vi "Database.Connect.vi"(8 "error in":errorcluster, 11 "Data in":T1) -> (0 "error out":errorcluster, 3 "Data out":T1)   [LabVIEW 2016]
doc: "Connect to database\n\nWabco 2017 All right reserved\nAuthor: maciej.szupienko@wabco-auto.com"
uses:
  Database.Data.ctl
  Database.Data.Sets.ctl
  Handler/Database.Handler.Data.Status.ctl
  Tools/Translator/Translator.Message.ctl
  Tools/EventLog/EventLog.EventSource.ctl
  Tools/EventLog/EventLog.New(array).vi
  Tools/EventLog/EventLog.CreateError(array).vi
  Tools/ErrorHandling/ErrorHandling.Create.vi
  Global/ApplicationGlobal.vi
  Tools/EventLog/EventLog.Buffer.vi
  Tools/EventLog/EventLog.File.ReadWrite.vi
  Tools/Tma.lib/string.llb/Join array to string.vi
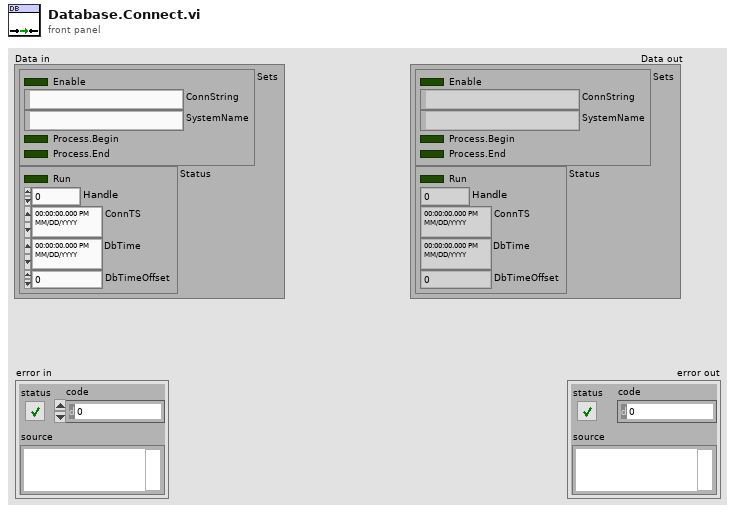
[diagram p1: front panel]
types:
  T1 = typedef "Database.Data.ctl" = cluster{"Sets":T2, "Status":T3}
  T2 = typedef "Database.Data.Sets.ctl" = cluster{"Enable":bool, "ConnString":string, "SystemName":string, "Process.Begin":bool, "Process.End":bool}
  T3 = typedef "Database.Handler.Data.Status.ctl" = cluster{"Run":bool, "Handle":i32, "ConnTS":timestamp, "DbTime":timestamp, "DbTimeOffset":dbl}
  T4 = typedef "EventLog.EventSource.ctl" = enum16{"All", "Gui", "Cache", "PLC1", "PLC2", "PLC3", "DB", "DB01", "DB02", "DB03", "DB04", "DB05", "DB06", "DB07", "DB08", "DB09", "DB10", "DB11", "DB12", "DB13", "DB14", "DB15", "DB16"}
  T5 = typedef "Translator.Message.ctl" = enum16{"-", "Event confirmed", "Log out", "Log in", "Shutdown", "Cancel", "Start", "Continue", "Stop", "On", "Off", "OK", "NOK", "NOK %s", "This", "Prev", "Home", "Work", "In progress...", "Missing", "Empty", "Hardware failure", "Initial", "Error %d >> %s", "Error %d >> %s >> %s", "Starting %s", "Quitting %s", "Configured", "Initializing", "Quitting", "Loading", "Running %s", "Stopped", "Summary", "Do you want to continue?", "Do you want to exit?", "Log out?", "System", "All", "IDLE", "Translating...%s", "Not found", "Alarm %s", "Run", "Skip", "Abort", "Repeat", "Please wait...", "Database disconnected", "Login to database successful", "Login to database failed: %d; %s", "Get process step data for %s", "Changeover off", "Changeover into %s", "Product %s | %s found in cache with status %d at previous station", "Product %s | %s found in database with status %d at previous station", "Product %s | %s not found in cache at previous station", "Product %s | %s not found in database at previous station", "Product %s | %s found in cache with status %d at this station (%d repetion)", "Product %s | %s found in database with status %d at this station (%d repetition)", "Product %s | %s not found in cache at this station", "Product %s | %s not found in database at this station", "Product %s | %s found in cache for component %s | %s", "Product %s | %s found in database for component %s | %s", "Product not found in cache for component %s | %s", "Product not found in database for component %s | %s", "Product %s | %s connected with component %s | %s (cache)", "Product %s | %s connected with component %s | %s (database)", "New data for %s | %s (cache)", "New data for %s | %s (database)", "File %s moved (cache)", "File %s deleted (cache)", "Msg %d >> %s", "PLC LifeBit Failure", "Reconnecting DB", "Reconnecting PLC", "Free disk space is below 1GB - contact technician", "Unable to check product status", "Product %s SN %s checked in DB", "Unable To check status from station %s"}
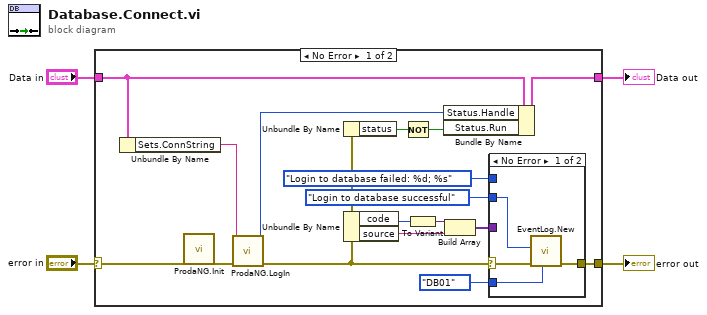
[diagram p0: block diagram]
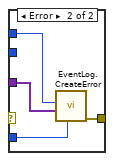
[diagram p2: hidden frame]
diagram:
  n1 = case shown="No Error" "error in" {
    selector: "error in" -> [w6 w31]
    tunnel: [w14 w31] -> w4
    tunnel: [w19 w30] -> w3
    tunnel: "Data in" -> [w18 w30]
    frame No Error {
      n2 = Unbundle By Name(w18) -> ("Sets.ConnString"=w8:string)
      n3 = call "ProdaNG.Init.vi"("error in (no error)"=w6) -> ("error out"=w5:errorcluster)  [unwired: 10 in]
      n4 = call "ProdaNG.LogIn.vi"("error in"=w5, "ConnectionString"=w8) -> ("error out"=w13:errorcluster, "dbHandle"=w9:i32)  [unwired: 7 in, 1 out]
      n5 = Unbundle By Name(w13) -> ("status"=w20:bool)
      n6 = Unbundle By Name(w13) -> ("code"=w17:i32, "source"=w15:string)
      n7 = Not(x=w20) -> (.not. x?=w21:bool)
      n8 = To Variant(anything=w17) -> (Variant=w16:variant)
      n9 = Bundle By Name(cluster=w18, "Status.Handle"=w9, "Status.Run"=w21) -> (w19:T1)
      n10 = Build Array(w16, w15) -> (w12:variant[])
      n11 = case shown="No Error" w13 {
        selector: w13 -> [w23 _]
        tunnel: [w25 w29] -> w14
        tunnel: w12 -> [_ w28]
        tunnel: Translator.Message."Login to database failed: %d; %s" ("Message (-)") -> [_ w27]
        tunnel: Translator.Message."Login to database successful" ("Message (-)") -> [w24 _]
        tunnel: EventLog.EventSource."DB01" ("Source (All)") -> [w22 w26]
        frame No Error {
          n12 = call-poly "EventLog.New.vi"("Source (All)"=w22, "error in (no error)"=w23, "Message (-)"=w24) -> ("error out"=w25:errorcluster)  [unwired: 7 in, 1 out]
        }
        frame Error {
          n13 = call-poly "EventLog.CreateError.vi"("Source (All)"=w26, "args"=w28, "Msg"=w27) -> ("error out"=w29:errorcluster)  [unwired: 7 in, 1 out]
        }
      }
    }
    frame Error {
    }
  }
  "error out" <- w4
  "Data out" <- w3
